vi "New Action.vi"(9 "View":i32[](array[numeric]) caption="View (Team Index, -1: empty)", 10 "Team Index":i32, 11 "AndrewF in":refnum<class "AndrewF.lvclass">) -> (0 "Replicated":refnum<class "Square.lvclass">, 1 "Direction":T2, 2 "Action":T1, 3 "AndrewF out":refnum<class "AndrewF.lvclass">)   [LabVIEW 2016, in "AndrewF.lvclass"]
uses:
  AndrewF.lvclass
  C:/Users/crwec/Desktop/Workspace/SquareBattle/Square/Square.lvclass
  Square/Square.lvclass
  Type Defs/Direction Enum.ctl
  Type Defs/Action Enum.ctl
  AndrewF.lvclass/AndrewF.ctl
  SubVIs/Read-Only Globals.vi
  SubVIs/Globals (private).vi
  Common/Common.lvlib
  Type Defs/SB Type Defs.lvlib
panel:
  # "NW\nN\nNE\nE\nSE\nS\nSW\nW"
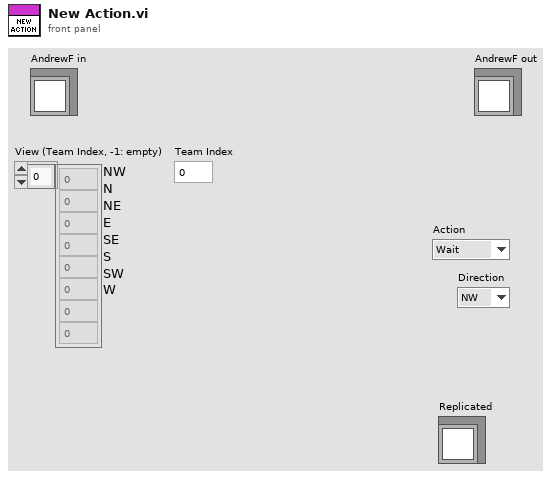
[diagram p1: front panel]
types:
  T1 = typedef "SB Type Defs.lvlib/Action Enum.ctl" = enum16{"Wait", "Move", "Attack", "Replicate"}
  T2 = typedef "SB Type Defs.lvlib/Direction Enum.ctl" = enum16{"NW", "N", "NE", "E", "SE", "S", "SW", "W"}
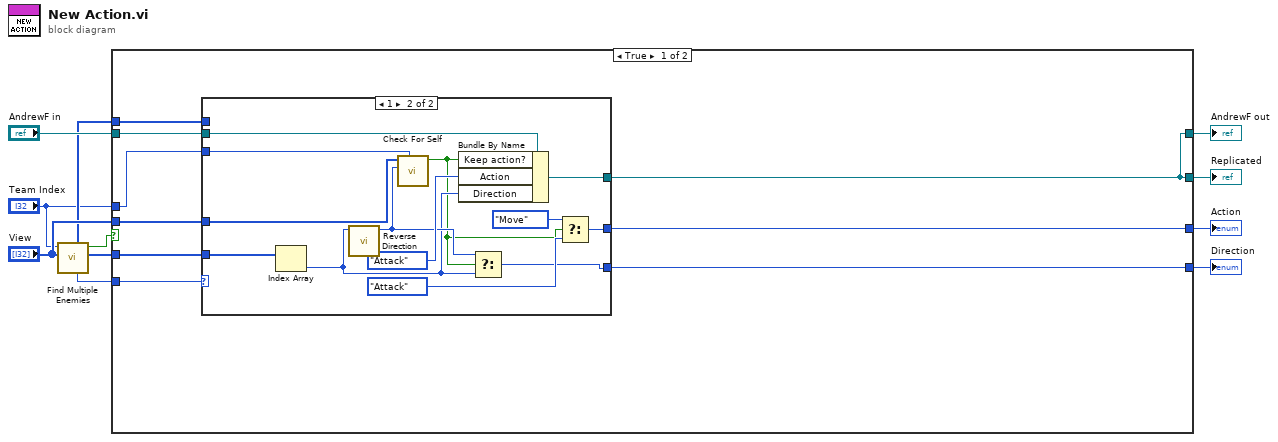
[diagram p0: block diagram]
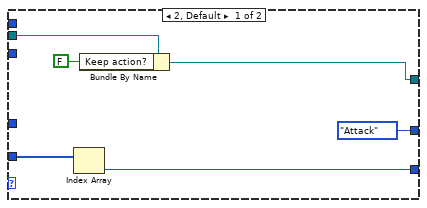
[diagram p2: hidden frame]
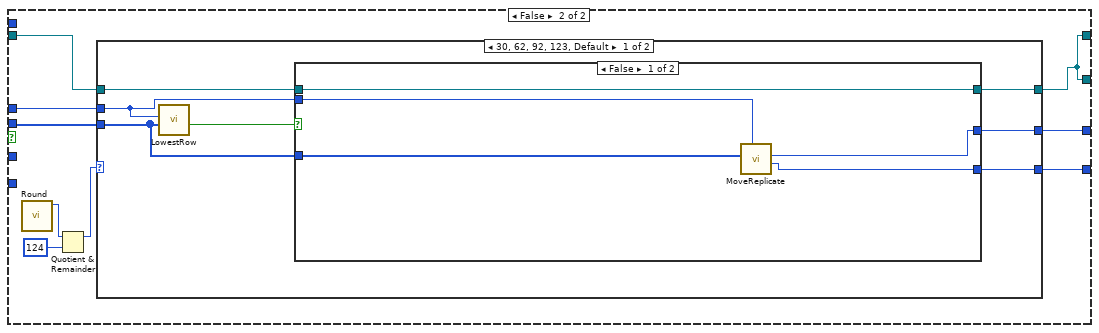
[diagram p3: hidden frame]
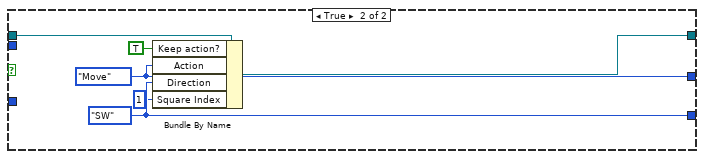
[diagram p4: hidden frame]
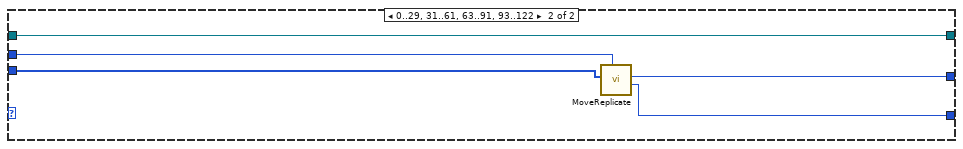
[diagram p5: hidden frame]
diagram:
  n1 = call "Find Multiple Enemies.vi"("View"="View", "Team Index"="Team Index") -> ("Direction"=w4:T2[], "Found Enemy?"=w2:bool, "How Many Enemies"=w3:i32, "Enemy"=w5:i32[])  [unwired: 6 in]
  n2 = case shown="True" w2 {
    tunnel: [w14 w40] -> w7
    tunnel: [w19 w46] -> w9
    tunnel: [w20 w48] -> w8
    tunnel: [w14 w40] -> w10
    tunnel: "AndrewF in" -> [w15 w41]
    tunnel: w3 -> [w18 _]
    tunnel: w4 -> [w17 _]
    tunnel: w5 -> [w16 _]
    tunnel: "View" -> [w13 w47]
    tunnel: "Team Index" -> [w12 w42]
    frame True {
      n3 = case shown="1" w18 {
        tunnel: [Action_Enum."Attack" ("Action") w34] -> w20
        tunnel: [w22 w29] -> w19
        tunnel: w17 -> [w23 w39]
        tunnel: w16 -> [_ _]
        tunnel: w15 -> [w26 w38]
        tunnel: [w25 w37] -> w14
        tunnel: w13 -> [_ w33]
        tunnel: w12 -> [_ w27]
        frame 2, Default {
          n4 = Index Array(array=w23) -> (element=w22:T2)  [unwired: 1 in]
          n5 = Bundle By Name(cluster=w26, "Keep action?"=FALSE) -> (w25:refnum<class "AndrewF.lvclass">)
        }
        frame 1 {
          n6 = Index Array(array=w39) -> (element=w30:T2)  [unwired: 1 in]
          n7 = call "Reverse Direction.vi"("Direction in"=w30) -> ("Reverse Direction"=w31:i32)  [unwired: 10 in]
          n8 = call "Check For Self.vi"("Team index"=w27, "Direction"=w31, "Map"=w33) -> ("Clear?"=w28:bool)  [unwired: 8 in]
          n9 = Bundle By Name(cluster=w38, "Keep action?"=w28, "Action"=Action_Enum."Attack", "Direction"=w30) -> (w37:refnum<class "AndrewF.lvclass">)
          n10 = Select(t=w31, s=w28, f=w30) -> (s? t:f=w29:i32)
          n11 = Select(t=Action_Enum."Move" ("Action"), s=w28, f=Action_Enum."Attack") -> (s? t:f=w34:T1)
        }
      }
    }
    frame False {
      n12 = call "Round.vi"() -> ("Round"=w45:i32)  [unwired: 11 in]
      n13 = Quotient & Remainder(x=w45, y=124) -> (x-y*floor(x/y)=w43:i32)  [unwired: 1 out]
      n14 = case shown="30, 62, 92, 123, Default" w43 {
        tunnel: [w55 w71] -> w48
        tunnel: w47 -> [w51 w69]
        tunnel: [w54 w70] -> w46
        tunnel: w42 -> [w49 w67]
        tunnel: w41 -> [w52 w68]
        tunnel: [w50 w68] -> w40
        frame 30, 62, 92, 123, Default {
          n15 = call "LowestRow.vi"("View"=w51, "Team Index"=w49) -> ("Is lowest"=w53:bool)  [unwired: 9 in]
          n16 = case shown="False" w53 {
            tunnel: [w59 w63] -> w55
            tunnel: [w58 w62] -> w54
            tunnel: w52 -> [w57 w66]
            tunnel: w51 -> [w60 _]
            tunnel: [w57 w65] -> w50
            tunnel: w49 -> [w56 _]
            frame False {
              n17 = call "MoveReplicate.vi"("Team Index"=w56, "View"=w60) -> ("Direction"=w58:T2, "Action"=w59:T1)  [unwired: 8 in]
            }
            frame True {
              w63 = Action_Enum."Move" ("f")
              w62 = Direction_Enum."SW" ("Direction")
              n18 = Bundle By Name(cluster=w66, "Keep action?"=TRUE, "Action"=w63, "Direction"=w62, "Square Index"=1) -> (w65:refnum<class "AndrewF.lvclass">)
            }
          }
        }
        frame 0..29, 31..61, 63..91, 93..122 {
          n19 = call "MoveReplicate.vi"("Team Index"=w67, "View"=w69) -> ("Direction"=w70:T2, "Action"=w71:T1)  [unwired: 8 in]
        }
      }
    }
  }
  "AndrewF out" <- w10
  "Action" <- w8
  "Direction" <- w9
  "Replicated" <- w7
